vi "Calculate Potting Data.vi"(8 "error in":errorcluster, 11 "Potting Procedure in":refnum<class "Potting Procedure.lvclass">) -> (0 "error out":errorcluster, 2 "Module Potting Data":T1[](array[typedef]), 3 "Potting Procedure out":refnum<class "Potting Procedure.lvclass">)   [LabVIEW 2011, in "Potting Procedure.lvclass"]
uses:
  Potting Procedure.lvclass
  Shared Components/SyringeTool Class/Type Definitions/Module Potting Data.ctl
  Shared Components/Vec3d Class/Vec3d Class.lvclass
  Shared Components/Utils/Type Definitions/3d Line.ctl
  Shared Components/Utils/Type Definitions/3d Point.ctl
  Potting Procedure.lvclass/Potting Procedure.ctl
  Shared Components/Gantry Class/Gantry Class.lvclass
  Shared Components/Config Manager Class/Type Definitions/Potting Surface Type.ctl
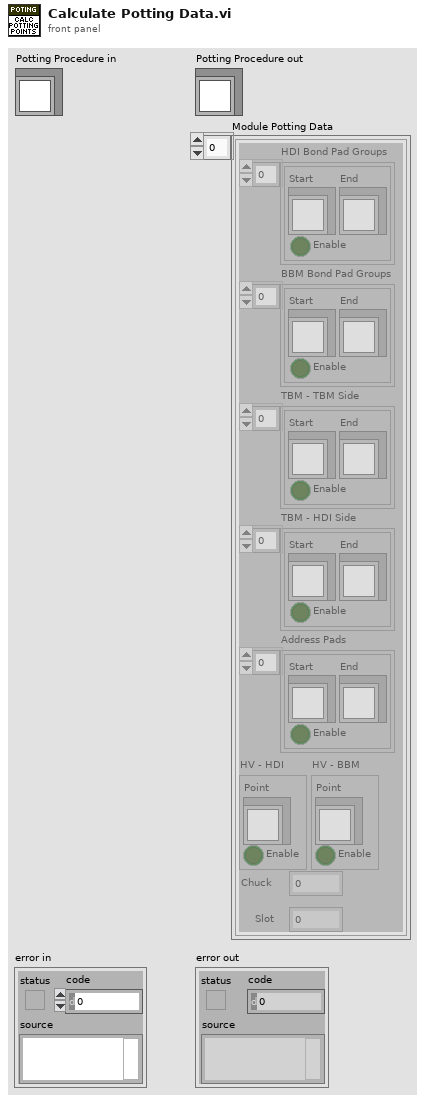
[diagram p1: front panel]
types:
  T1 = typedef "Module Potting Data.ctl" = cluster{"HDI Bond Pad Groups":T2[], "BBM Bond Pad Groups":T2[], "TBM - TBM Side":T2[], "TBM - HDI Side":T2[], "Address Pads":T2[], "Chuck":i32, "Slot":i32, "HV - HDI":T3, "HV - BBM":T3}
  T2 = typedef "3d Line.ctl" = cluster{"Start":refnum<class "Vec3d Class.lvclass">, "End":refnum<class "Vec3d Class.lvclass">, "Enable":bool}
  T3 = typedef "3d Point.ctl" = cluster{"Point":refnum<class "Vec3d Class.lvclass">, "Enable":bool}
  T4 = typedef "Potting Surface Type.ctl" = enum16{"default", "hdi_edge_pads", "bbm_edge_pads", "address_pads"}
  T5 = typedef "Inspect Modules - Module.ctl" = cluster{"TBM-TBM":T6, "TBM-HDI":T6, "Address Pads":T6, "HDI Bond Pad References":T10[], "BBM Bond Pad References":T10[], "HV-HDI":T10, "HV-BBM":T10, "Chuck":i32, "Slot":i32, "Potting Selection":cluster{"HDI Bond Pads":bool[], "BBM Bond Pads":bool[], "TBM Inner":cluster{"Top":bool, "Left":bool, "Bottom":bool, "Right":bool}, "TBM Outer":cluster{"Top":bool, "Left":bool, "Bottom":bool, "Right":bool}, "Address Pads":cluster{"Top":bool, "Bottom":bool}, "High Voltage":cluster{"HDI":bool, "BBM":bool}}}
  T6 = typedef "Multi-Fiducial Image.ctl" = cluster{"Fiducial Image":T7, "Fiducials":cluster{"Selected Fiducial":T9, "fiducial name":string}[]}
  T7 = typedef "Physical Image.ctl" = cluster{"Image Position":refnum<class "Vec3d Class.lvclass">, "Image Reference":T8, "Field of View":cluster{"x(mm)":dbl, "y(mm)":dbl}}
  T8 = typedef "IMAQ Image.ctl" = refnum<image>
  T9 = typedef "Fiducial with Source.ctl" = cluster{"Fiducial Image Coordinate":refnum<class "Vec3d Class.lvclass">, "Fiducial Source":enum16{"Pattern Recognition", "User", "Error", "Default"}}
  T10 = typedef "Fiducial Image.ctl" = cluster{"Fiducial Image":T7, "Selected Fiducial":T9, "fiducial name":string}
  T11 = cluster{"Top":bool, "Left":bool, "Bottom":bool, "Right":bool}
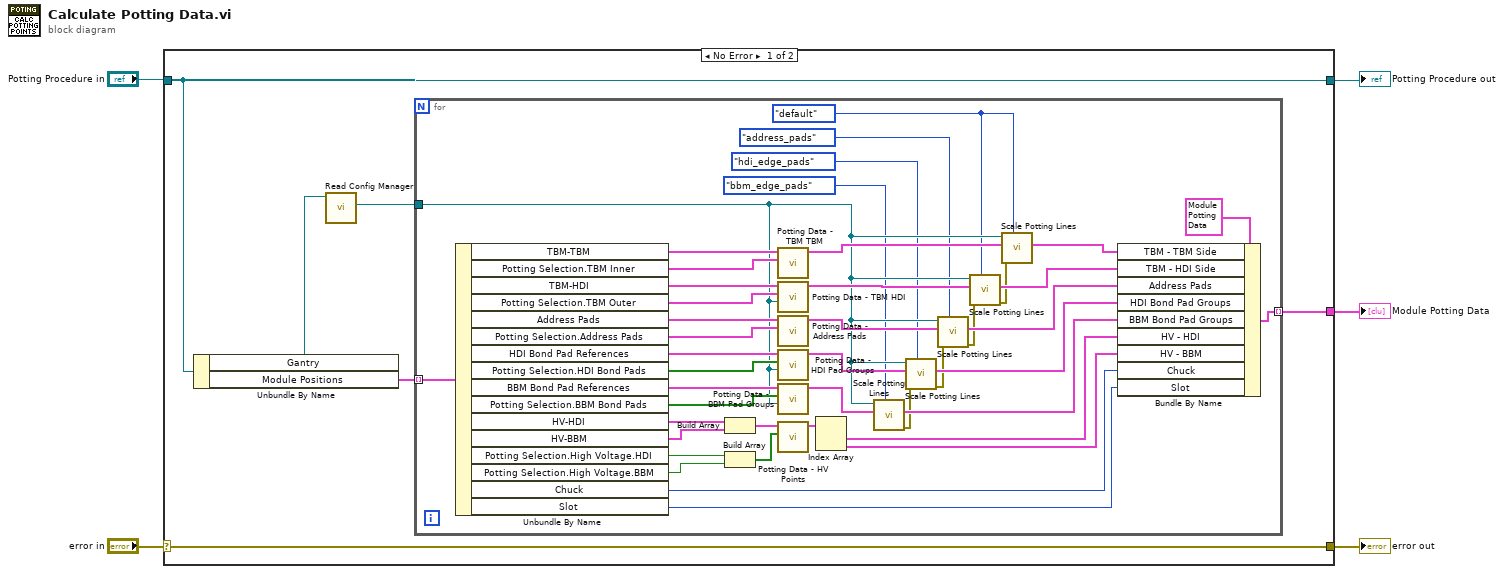
[diagram p0: block diagram]
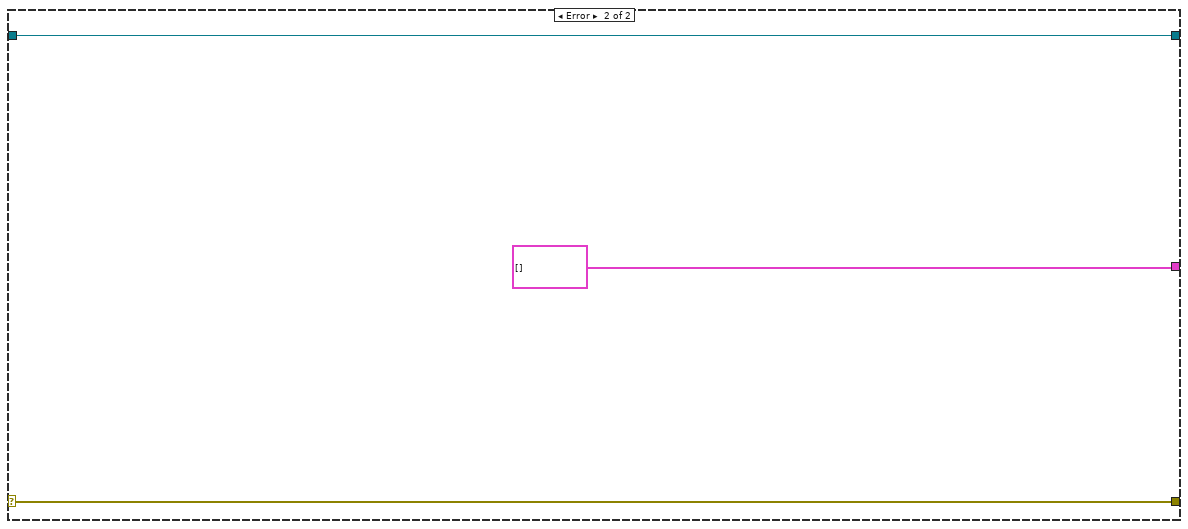
[diagram p2: hidden frame]
diagram:
  n1 = case shown="No Error" "error in" {
    selector: "error in" -> [w11 w57]
    tunnel: [w11 w57] -> w3
    tunnel: "Potting Procedure in" -> [w7 w56]
    tunnel: [w7 w56] -> w2
    tunnel: [w6 T1[] []] -> w1
    frame No Error {
      n2 = Unbundle By Name(w7) -> ("Gantry"=w9:refnum<class "Gantry Class.lvclass">, "Module Positions"=w10:T5[])
      n3 = call-dynamic "Read Config Manager.vi"("Gantry in"=w9) -> ("Config Manager"=w8:refnum<class "Config Manager Class.lvclass">)  [unwired: 8 in, 2 out]
      n4 = for {
        tunnel: w10 -> [w49] mode=indexing
        tunnel: w8 -> [w20]
        tunnel: [w40] -> w6 mode=indexing
        w19 = Potting_Surface_Type."default" ("Potting Surface Type")
        n5 = Unbundle By Name(w49) -> ("TBM-TBM"=w54:T6, "Potting Selection.TBM Inner"=w53:T11, "TBM-HDI"=w52:T6, "Potting Selection.TBM Outer"=w51:T11, "Address Pads"=w48:T6, "Potting Selection.Address Pads"=w50:cluster{"Top":bool, "Bottom":bool}, "HDI Bond Pad References"=w47:T10[], "Potting Selection.HDI Bond Pads"=w46:bool[], "BBM Bond Pad References"=w45:T10[], "Potting Selection.BBM Bond Pads"=w44:bool[], "HV-HDI"=w39:T10, "HV-BBM"=w38:T10, "Potting Selection.High Voltage.HDI"=w36:bool, "Potting Selection.High Voltage.BBM"=w35:bool, "Chuck"=w42:i32, "Slot"=w41:i32)
        n6 = Build Array(w39, w38) -> (w37:T10[])
        n7 = Build Array(w36, w35) -> (w34:bool[])
        n8 = call "Potting Data - TBM TBM.vi"("TBM-TBM Selection"=w53, "TBM-TBM Data"=w54) -> ("Potting Lines"=w33:T2[])  [unwired: 8 in, 1 out]
        n9 = call "Potting Data - TBM HDI.vi"("Config Manager"=w20, "TBM-HDI Selection"=w51, "TBM-HDI Data"=w52) -> ("Potting Lines"=w32:T2[])  [unwired: 7 in, 1 out]
        n10 = call "Potting Data - Address Pads.vi"("Address Pads Selection"=w50, "Address Pads Data"=w48) -> ("Potting Lines"=w31:T2[])  [unwired: 8 in, 1 out]
        n11 = call "Potting Data - HDI Pad Groups.vi"("Config Manager"=w20, "Potting Selection HDI Bond Pads"=w46, "HDI Bond Pad References"=w47) -> ("Potting Lines"=w30:T2[])  [unwired: 7 in, 1 out]
        n12 = call "Potting Data - BBM Pad Groups.vi"("Config Manager"=w20, "Potting Selection BBM Bond Pads"=w44, "BBM Bond Pad References"=w45) -> ("Potting Lines"=w29:T2[])  [unwired: 7 in, 1 out]
        n13 = call "Potting Data - HV Points.vi"("HV Point Selection"=w34, "HV Point Data"=w37) -> ("HV Potting Points"=w28:T3[])  [unwired: 8 in, 1 out]
        n14 = Index Array(array=w28) -> (element #1=w27:T3, element #2=w26:T3)  [unwired: 2 in]
        n15 = call "Scale Potting Lines.vi"("Potting Surface Type"=Potting_Surface_Type."bbm_edge_pads", "Potting Lines"=w29, "Config Manager"=w20) -> ("error out"=w17:errorcluster, "Potting Lines Scaled"=w25:T2[])  [unwired: 7 in]
        n16 = call "Scale Potting Lines.vi"("Potting Surface Type"=Potting_Surface_Type."hdi_edge_pads", "error in"=w17, "Potting Lines"=w30, "Config Manager"=w20) -> ("error out"=w16:errorcluster, "Potting Lines Scaled"=w24:T2[])  [unwired: 6 in]
        n17 = call "Scale Potting Lines.vi"("Potting Surface Type"=Potting_Surface_Type."address_pads", "error in"=w16, "Potting Lines"=w31, "Config Manager"=w20) -> ("error out"=w15:errorcluster, "Potting Lines Scaled"=w23:T2[])  [unwired: 6 in]
        n18 = call "Scale Potting Lines.vi"("Potting Surface Type"=w19, "error in"=w15, "Potting Lines"=w32, "Config Manager"=w20) -> ("error out"=w14:errorcluster, "Potting Lines Scaled"=w22:T2[])  [unwired: 6 in]
        n19 = call "Scale Potting Lines.vi"("Potting Surface Type"=w19, "error in"=w14, "Potting Lines"=w33, "Config Manager"=w20) -> ("Potting Lines Scaled"=w21:T2[])  [unwired: 6 in, 1 out]
        n20 = Bundle By Name(cluster=T1 {"HDI Bond Pad Groups"=[], "BBM Bond Pad Groups"=[], "TBM - TBM Side"=[], "TBM - HDI Side"=[], "Address Pads"=[], "Chuck"=0, "Slot"=0, "HV - HDI"={"Point"=refnum, "Enable"=FALSE}, "HV - BBM"={"Point"=refnum, "Enable"=FALSE}} ("Module Potting Data"), "TBM - TBM Side"=w21, "TBM - HDI Side"=w22, "Address Pads"=w23, "HDI Bond Pad Groups"=w24, "BBM Bond Pad Groups"=w25, "HV - HDI"=w27, "HV - BBM"=w26, "Chuck"=w42, "Slot"=w41) -> (w40:T1)
      }
    }
    frame Error {
    }
  }
  "error out" <- w3
  "Potting Procedure out" <- w2
  "Module Potting Data" <- w1
